vi "Set Grating.vi"(8 "error in (no error)":errorcluster, 10 "Grating ID":i32, 11 "VISA resource name":refnum<visa-resource-name>) -> (0 "error out":errorcluster, 3 "VISA resource name out":refnum<visa-resource-name>, 4 "read buffer":string)   [LabVIEW 2019, in "SpectraPro.lvlib"]
uses:
  SpectraPro.lvlib
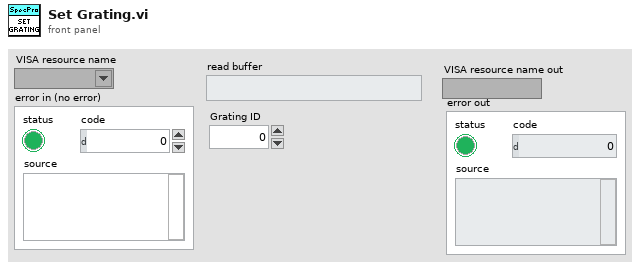
[diagram p1: front panel]
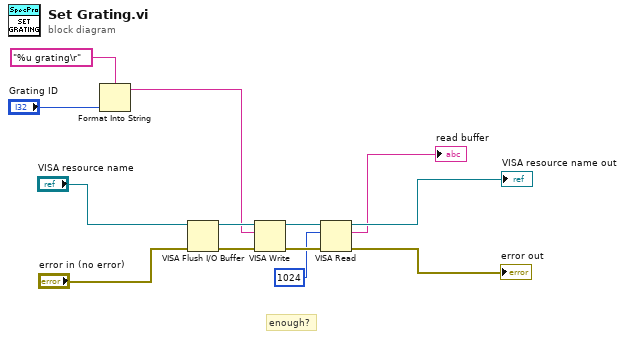
[diagram p0: block diagram]
diagram:
  # "enough?"
  n1 = Format Into String(format string="%u grating\r", "Grating ID") -> (resulting string=w1:string)  [unwired: 2 in, 1 out]
  n2 = VISA Flush I/O Buffer(VISA resource name="VISA resource name", error in (no error)="error in (no error)") -> (VISA resource name out=w7:refnum<visa-resource-name>, error out=w8:errorcluster)  [unwired: 1 in]
  n3 = VISA Write(VISA resource name=w7, write buffer=w1, error in (no error)=w8) -> (VISA resource name out=w10:refnum<visa-resource-name>, error out=w11:errorcluster)  [unwired: 1 out]
  n4 = VISA Read(VISA resource name=w10, byte count=u32 1024, error in (no error)=w11) -> (VISA resource name out=→"VISA resource name out":refnum<visa-resource-name>, read buffer=→"read buffer":string, error out=→"error out":errorcluster)  [unwired: 1 out]
